vi "Build sinusoid.vi"(0 "t":dbl[](array[numeric]), 5 "t2":dbl[](array[numeric]), 9 "phase":dbl, 11 "amplitude":dbl, 12 "frequency":dbl, 13 "dfreq":dbl, 14 "damp":dbl) -> (4 "signal out":dbl[](array[numeric]), 10 "last phase":dbl, 15 "last amplitude":dbl)   [LabVIEW 2012]
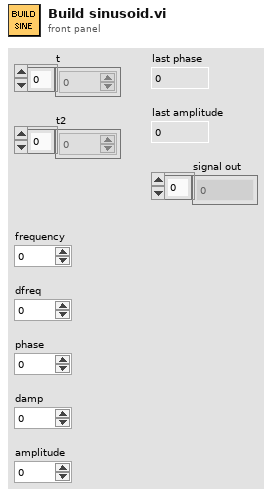
[diagram p1: front panel]
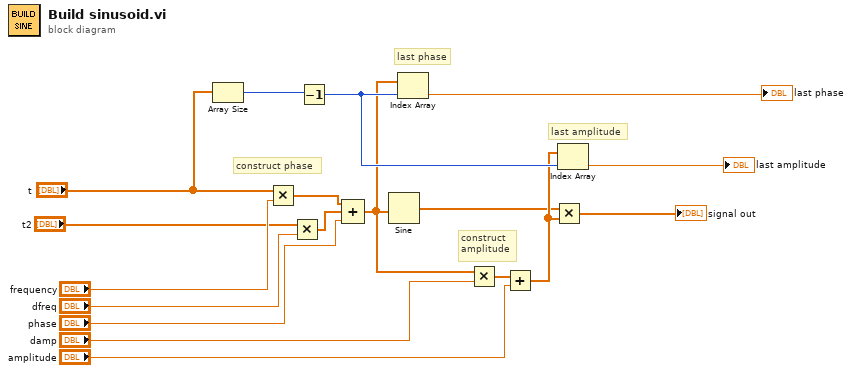
[diagram p0: block diagram]
diagram:
  # "last amplitude"
  # "construct\namplitude"
  # "last phase"
  # "construct phase"
  n1 = Array Size(array="t") -> (size(s)=w1:i32)
  n2 = Multiply(x="t", y="frequency") -> (x*y=w3:dbl[])
  n3 = Multiply(x="t2", y="dfreq") -> (x*y=w2:dbl[])
  n4 = Decrement(x=w1) -> (x-1=w8:i32)
  n5 = Compound Arithmetic op=ADD(w3, w2, "phase") -> (w6:dbl[])
  n6 = Sine(x=w6) -> (sin(x)=w5:dbl[])
  n7 = Index Array(array=w6, index=w8) -> (element=→"last phase":dbl)
  n8 = Multiply(x=w6, y="damp") -> (x*y=w4:dbl[])
  n9 = Add(x=w4, y="amplitude") -> (x+y=w7:dbl[])
  n10 = Multiply(x=w5, y=w7) -> (x*y=→"signal out":dbl[])
  n11 = Index Array(array=w7, index=w8) -> (element=→"last amplitude":dbl)
